vi "Rotate Points 2.vi"(10 "Rotation Matrix":T2, 11 "Positions":T1[](array[typedef])=[{"X"=649.0, "Y"=640.0, "Z"=665.0}, {"X"=682.0, "Y"=-795.0, "Z"=504.0}, {"X"=-784.0, "Y"=533.0, "Z"=-524.0}, {"X"=-644.0, "Y"=584.0, "Z"=-595.0}, {"X"=-588.0, "Y"=-843.0, "Z"=648.0}, {"X"=-30.0, "Y"=6.0, "Z"=44.0}, {"X"=-674.0, "Y"=560.0, "Z"=763.0}, {"X"=500.0, "Y"=723.0, "Z"=-460.0}, {"X"=609.0, "Y"=671.0, "Z"=-379.0}, {"X"=-555.0, "Y"=-800.0, "Z"=653.0}, {"X"=-675.0, "Y"=-892.0, "Z"=-343.0}, {"X"=697.0, "Y"=-426.0, "Z"=-610.0}, {"X"=578.0, "Y"=704.0, "Z"=681.0}, {"X"=493.0, "Y"=664.0, "Z"=-388.0}, {"X"=-671.0, "Y"=-858.0, "Z"=530.0}, {"X"=-667.0, "Y"=343.0, "Z"=800.0}, {"X"=571.0, "Y"=-461.0, "Z"=-707.0}, {"X"=-138.0, "Y"=-166.0, "Z"=112.0}, {"X"=-889.0, "Y"=563.0, "Z"=-600.0}, {"X"=646.0, "Y"=-828.0, "Z"=498.0}, {"X"=640.0, "Y"=759.0, "Z"=510.0}, {"X"=-630.0, "Y"=509.0, "Z"=768.0}, {"X"=-681.0, "Y"=-892.0, "Z"=-333.0}, {"X"=673.0, "Y"=-379.0, "Z"=-804.0}, {"X"=-742.0, "Y"=-814.0, "Z"=-386.0}, {"X"=577.0, "Y"=-820.0, "Z"=562.0}]) -> (3 "Rotated":T1[](array[typedef]))   [LabVIEW 2020]
uses:
  Vec3.ctl
  <vilib>/Analysis/Matrix/Datatypes/RealMatrix.ctl
  <vilib>/Analysis/Matrix/Numeric/Conversions/Array To Matrix - RA.vi
  <vilib>/Analysis/Matrix/Numeric/Multiply/Multiply - RM,RM.vi
  <vilib>/Analysis/Matrix/Numeric/Conversions/Matrix To Array - RM.vi
  <vilib>/Analysis/Matrix/NI_Matrix.lvlib
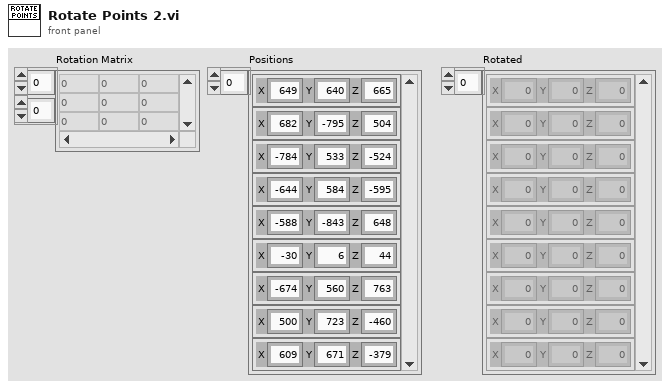
[diagram p1: front panel]
types:
  T1 = typedef "Vec3.ctl" = cluster{"X":dbl, "Y":dbl, "Z":dbl}
  T2 = typedef "NI_Matrix.lvlib/RealMatrix.ctl" = dbl[][]
  T3 = cluster{"Real 2D Array[0]":dbl, "Real 2D Array[1]":dbl, "Real 2D Array[2]":dbl}
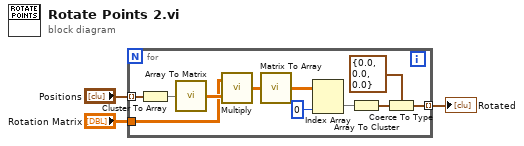
[diagram p0: block diagram]
diagram:
  n1 = for {
    tunnel: "Positions" -> [w14] mode=indexing
    tunnel: [w4] -> w1 mode=indexing
    tunnel: "Rotation Matrix" -> [w10]
    n2 = Cluster To Array(cluster=w14) -> (array=w13:dbl[])
    n3 = call-poly <vilib>:"Array To Matrix.vi"("Real 1D Array"=w13) -> ("Real Matrix (Column Vector)"=w11:T2)
    n4 = call-poly <vilib>:"Multiply.vi"("Real Matrix B"=w11, "Real Matrix A"=w10) -> ("A * B"=w12:T2)
    n5 = call-poly <vilib>:"Matrix To Array.vi"("Real Matrix"=w12) -> ("Real 2D Array"=w9:dbl[][])
    n6 = Index Array(array=w9, index (col)=0 ("disabled index (col)")) -> (element=w7:dbl[])  [unwired: 1 in]
    n7 = Array To Cluster(array=w7) -> (cluster=w6:T3)
    n8 = Coerce To Type(0:w6, 1:T1 {"X"=0.0, "Y"=0.0, "Z"=0.0} ("Position")) -> (2:w4:T1)
  }
  "Rotated" <- w1
